vi "Or-Opt(Zobolas) Neighborhood.vi"(8 "w":i32, 9 "y":i32, 10 "Generate Random Indices?":bool, 11 "C'":u16[](array[numeric])) -> (3 "Chromosome Out":u16[](array[numeric]))   [LabVIEW 2013]
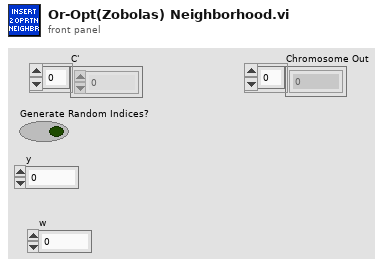
[diagram p1: front panel]
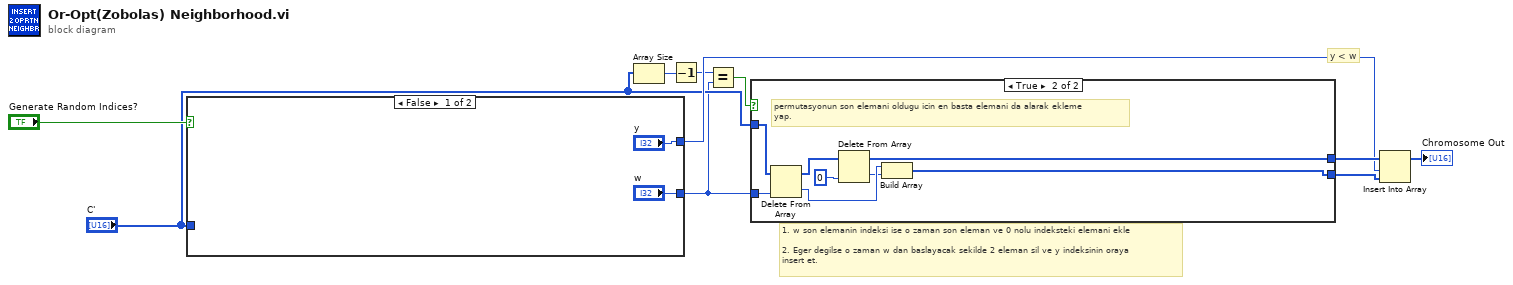
[diagram p0: block diagram]
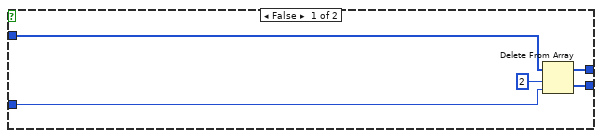
[diagram p2: hidden frame]
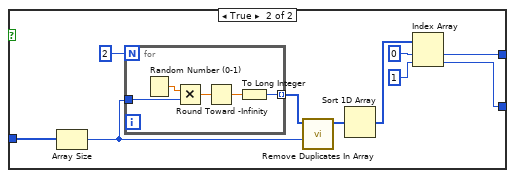
[diagram p3: hidden frame]
diagram:
  # "1. w son elemanin indeksi ise o zaman son eleman ve 0 nolu indeksteki elemani ekle\n\n2. Eger degilse o zaman w dan baslayacak sekilde 2 eleman sil ve y indeksinin oraya\ninsert et."
  # "y < w"
  n1 = case shown="False" "Generate Random Indices?" {
    tunnel: "C'" -> [_ w22]
    tunnel: ["w" w13] -> w2
    tunnel: ["y" w14] -> w8
    frame False {
    }
    frame True {
      n2 = Array Size(array=w22) -> (size(s)=w19:i32)
      n3 = for {
        N: 2 -> [_]
        tunnel: w19 -> [w26]
        tunnel: [w23] -> w20 mode=indexing
        n4 = Random Number (0-1)() -> (number: 0 to 1=w27:dbl)
        n5 = Multiply(x=w27, y=w26) -> (x*y=w25:dbl)
        n6 = Round Toward -Infinity(1:w25) -> (0:w24:dbl)
        n7 = To Long Integer(number=w24) -> (32bit integer=w23:i32)
      }
      n8 = call "Remove Duplicates In Array.vi"("Max Index Bound"=w19, "Random Numbers Array"=w20) -> ("Random Numbers Array without Duplicates"=w16:i32[])  [unwired: 9 in]
      n9 = Sort 1D Array(array=w16) -> (sorted array=w15:i32[])
      n10 = Index Array(array=w15, index #1=0 ("index"), index #2=1 ("index")) -> (element #1=w14:i32, element #2=w13:i32)
    }
  }
  n11 = Array Size(array="C'") -> (size(s)=w4:i32)
  n12 = Decrement(x=w4) -> (x-1=w3:i32)
  n13 = Equal?(x=w3, y=w2) -> (x = y?=w1:bool)
  n14 = case shown="True" w1 {
    tunnel: "C'" -> [w32 w40]
    tunnel: [w31 w36] -> w9
    tunnel: w2 -> [w30 w39]
    tunnel: [w29 w33] -> w7
    frame False {
      n15 = Delete From Array(array=w32, length=2, index=w30) -> (deleted portion=w29:u16[], array with subset deleted=w31:u16[])
    }
    frame True {
      # "permutasyonun son elemani oldugu icin en basta elemani da alarak ekleme\nyap."
      n16 = Delete From Array(array=w40, index=w39) -> (deleted portion=w35:u16, array with subset deleted=w38:u16[])  [unwired: 1 in]
      n17 = Delete From Array(array=w38, index=0) -> (deleted portion=w34:u16, array with subset deleted=w36:u16[])  [unwired: 1 in]
      n18 = Build Array(w35, w34) -> (w33:u16[])
    }
  }
  n19 = Insert Into Array(array=w9, index=w8, new element=w7) -> (→"Chromosome Out":u16[])
